vi "LVClass_Pupil ctor from Zernike pupil.vi"(0 "Pupil (const)":refnum<class "Pupil.lvclass">, 5 "Dimensions_um":T2={"Size"={"X"=1, "Y"=2}, "Step"={"X"=3.0, "Y"=4.0}}, 7 "center":T1, 9 "rayon":sgl, 11 "error constant":errorcluster) -> (4 "Pupil (new)":refnum<class "Pupil.lvclass">, 15 "error IO":errorcluster)   [LabVIEW 2020, in "Pupil.lvclass"]
doc: "Circular Pupil constructor from dimensions, steps and circle shape.\n\n--------------------------------------------------------------------------------\n\n<B>PupilIn</B> : Constant Pointer to Pupil object.\n<B>PupilOut</B> : Pointer to Pupil object.\n<B>step</B> : Step x and y between the subpupils (um).\n<B>dimensions</B> : Pupil array dimensions (width, height).\n<B>center</B> : Center of the circle shape (um).\n<B>radius</B> : Radius of the circle shape (um).\n<B>ErrorIn</B> : Error\n<B>ErrorOut</B> : Error\n\n--------------------------------------------------------------------------------"
uses:
  Pupil.lvclass
  General dimensions definition.ctl
  Point2D.ctl
  Point2Df.ctl
  Handle creation.ctl
  Pupil.lvclass/Pupil.ctl
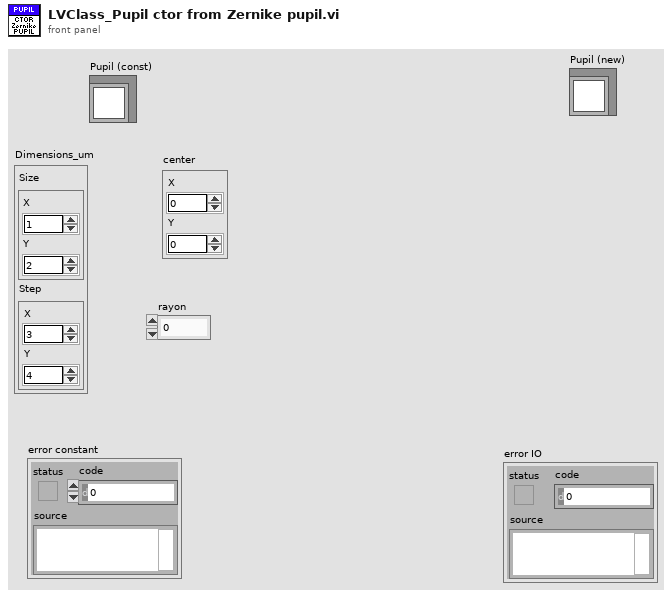
[diagram p1: front panel]
types:
  T1 = typedef "Point2Df.ctl" = cluster{"X":sgl, "Y":sgl}
  T2 = typedef "General dimensions definition.ctl" = cluster{"Size":T3, "Step":T1}
  T3 = typedef "Point2D.ctl" = cluster{"X":u32, "Y":u32}
  T4 = typedef "Handle creation.ctl" = enum16{"By ctor", "By write function"}
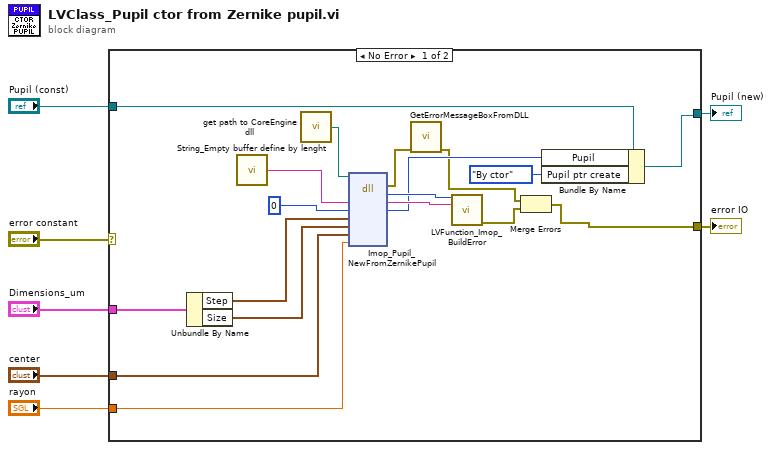
[diagram p0: block diagram]
diagram:
  n1 = case shown="No Error" "error constant" {
    selector: "error constant" -> [_ w27]
    tunnel: [w8 w27] -> w6
    tunnel: [w18 w26] -> w4
    tunnel: "Pupil (const)" -> [w19 w26]
    tunnel: "Dimensions_um" -> [w15 _]
    tunnel: "center" -> [w13 _]
    tunnel: "rayon" -> [w12 _]
    frame No Error {
      n2 = Unbundle By Name(w15) -> ("Step"=w11:T1, "Size"=w14:T3)
      n3 = call "String_Empty buffer define by lenght.vi"() -> ("Empty buffer"=w25:string)  [unwired: 1 in]
      n4 = call "get path to CoreEngine dll.vi"() -> ("path to wavekit library"=w22:path)  [unwired: 14 in, 1 out]
      n5 = dll-call lib="D:/soft/HASO_v3/SVN_trunk/ImOpCoreEngine4_LV2011/DLLs/c_interface_vc100.dll" fn="Imop_Pupil_NewFromZernikePupil"(path in=w22, "message"=w25, "Pupil"=0, "step"=w11, "Size"=w14, "center"=w13, "radius"=w12) -> (error out=w21:errorcluster, "return type"=w23:i32, "message"=w24:string, "Pupil"=w17:i64)  [unwired: 6 in, 1 out]
      n6 = call "GetErrorMessageBoxFromDLL.vi"("error IN"=w21) -> ("error OUT"=w10:errorcluster)  [unwired: 10 in]
      n7 = call "LVFunction_Imop_BuildError.vi"("code"=w23, "String to Prepend to source (\"\")"=w24) -> ("error out"=w9:errorcluster)  [unwired: 13 in]
      n8 = Merge Errors(w10, w9) -> (w8:errorcluster)
      n9 = Bundle By Name(cluster=w19, "Pupil"=w17, "Pupil ptr create"=Handle_creation."By ctor") -> (w18:refnum<class "Pupil.lvclass">)
    }
    frame Error {
    }
  }
  "error IO" <- w6
  "Pupil (new)" <- w4
